vi "ReadData.vi"(8 "error in (no error)":errorcluster, 10 "LogicName":string, 11 "PLC_Module in":refnum<class "PLC_Module.lvclass">) -> (0 "error out":errorcluster, 1 "plc error":errorcluster, 2 "Data":variant, 3 "PLC_Module out":refnum<class "PLC_Module.lvclass">)   [LabVIEW 2025, in "PLC_Module.lvlib" / "PLC_Module.lvclass"]
uses:
  PLC_Module.lvclass
  PLC_Module.lvclass/PLC_Module.ctl
  PLC_Abstr/PLC_Abstr Messages/Read Data Msg/Read Data Msg.lvclass/Read Data Msg.ctl
  <vilib>/ActorFramework/Message Enqueuer/Message Enqueuer.lvclass/Message Enqueuer.ctl
  Read Configuration.vi
  Read Connect.vi
  <vilib>/ActorFramework/Message Enqueuer/Enqueue.vi
  PLC_Abstr/PLC_Abstr Messages/Read Data Msg/Read Data Msg.lvclass
  C:/Program Files (x86)/National Instruments/LabVIEW 2025/vi.lib/ActorFramework/Message/Message.lvclass
  <vilib>/ActorFramework/Message Priority Queue/Priority Enqueue.vi
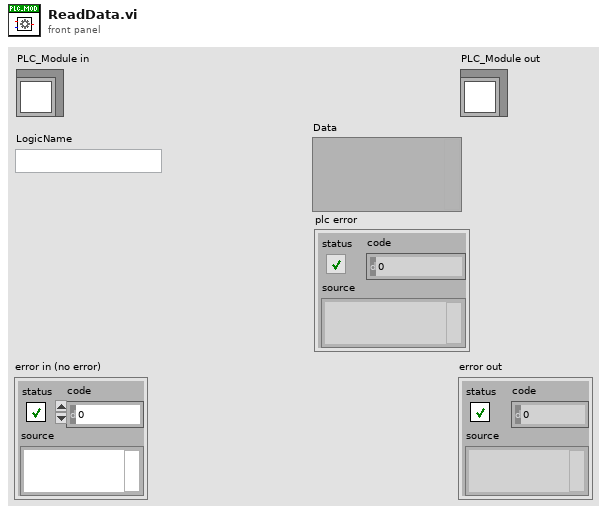
[diagram p1: front panel]
types:
  T1 = typedef "PLC_Module.lvlib/PLC_Module.lvclass/PLC_Data_Config.ctl" = map{string, cluster{"Config":T2, "Get Value":string, "Set Value":string}}
  T2 = typedef "PLC_Module.lvlib/PLC_Module.lvclass/PLC_Data.ctl" = cluster{"Address":string, "Direction":enum16{"PC->PLC", "PLC->PC"}, "DataType":T3, "Description":string}
  T3 = typedef "PLC_Module.lvlib/PLC_Module.lvclass/PLC_Data_Type.ctl" = enum16{"Boolean", "Single Float", "U8", "U32", "U32_Array", "String"}
  T4 = cluster{"Config":T2, "Get Value":string, "Set Value":string}
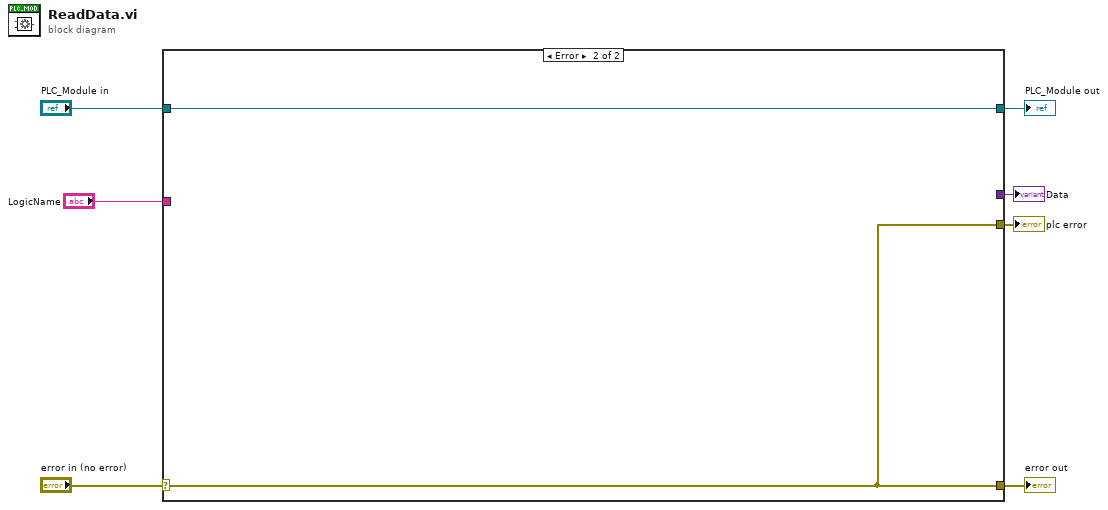
[diagram p0: block diagram]
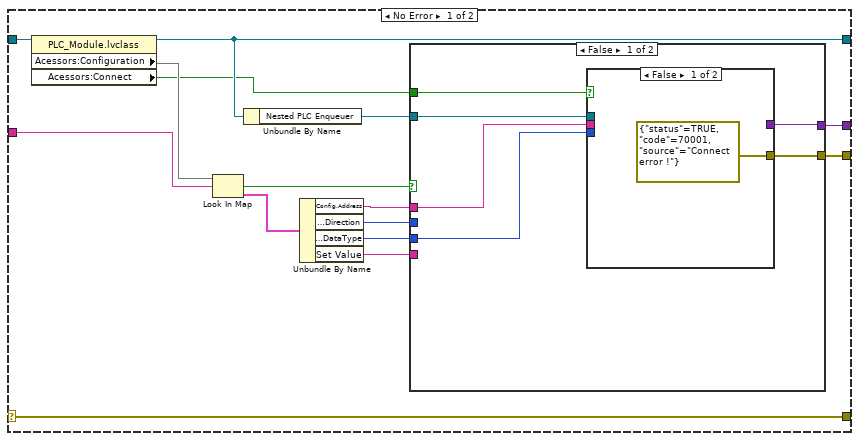
[diagram p2: hidden frame]
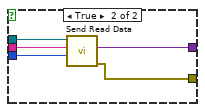
[diagram p3: hidden frame]
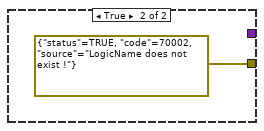
[diagram p4: hidden frame]
diagram:
  n1 = case shown="Error" "error in (no error)" {
    selector: "error in (no error)" -> [w22 w36]
    tunnel: [w22 w36] -> w6
    tunnel: [w18 w37] -> w4
    tunnel: "PLC_Module in" -> [w21 w37]
    tunnel: "LogicName" -> [w19 _]
    tunnel: [w10 _] -> w2
    tunnel: [w8 w36] -> w1
    frame No Error {
      n2 = property class="PLC_Module.lvclass"(reference=w21) -> (reference out=w18:refnum<class "PLC_Module.lvclass">, "Acessors:Configuration"=w20:T1, "Acessors:Connect"=w9:bool)  [unwired: 1 in, 1 out]
      n3 = Look In Map(map=w20, key=w19) -> (key not found?=w16:bool, value=w15:T4)  [unwired: 1 in]
      n4 = Unbundle By Name(w18) -> ("Nested PLC Enqueuer"=w17:refnum<class "Message Enqueuer.lvclass">)
      n5 = Unbundle By Name(w15) -> ("Config.Address"=w14:string, "Config.Direction"=w13:enum16{"PC->PLC", "PLC->PC"}, "Config.DataType"=w12:T3, "Set Value"=w11:string)
      n6 = case shown="False" w16 {
        tunnel: w17 -> [w28 _]
        tunnel: w14 -> [w26 _]
        tunnel: w13 -> [_ _]
        tunnel: w12 -> [w25 _]
        tunnel: w11 -> [_ _]
        tunnel: [w27 _] -> w10
        tunnel: w9 -> [w24 _]
        tunnel: [w23 errorcluster {"status"=TRUE, "code"=70002, "source"="LogicName does not exist !"} ("error out")] -> w8
        frame False {
          n7 = case shown="False" w24 {
            tunnel: w28 -> [_ w34]
            tunnel: [_ w31] -> w27
            tunnel: w26 -> [_ w33]
            tunnel: w25 -> [_ w32]
            tunnel: [errorcluster {"status"=TRUE, "code"=70001, "source"="Connect error !"} ("error out") w30] -> w23
            frame False {
            }
            frame True {
              n8 = call "Send Read Data.vi"("Data Type"=w32, "Address"=w33, "Message Enqueuer"=w34) -> ("error out"=w30:errorcluster, "Data"=w31:variant)  [unwired: 6 in, 1 out]
            }
          }
        }
        frame True {
        }
      }
    }
    frame Error {
    }
  }
  "error out" <- w6
  "PLC_Module out" <- w4
  "Data" <- w2
  "plc error" <- w1
